vi "Inst_K2002.vi"(8 "error in":errorcluster, 10 "All Message Queues in":T1, 11 "Prueba31 in":refnum<class "Prueba05.lvclass">) -> (0 "error out":errorcluster)   [LabVIEW 2019, in "Prueba05.lvclass"]
uses:
  Prueba05.lvclass
  QMH/Message Queue/All Message Queues.ctl
  QMH/Message Queue/Message Cluster.ctl
  Prueba05.lvclass/Prueba05.ctl
  <vilib>/Utility/error.llb/Error Cluster From Error Code.vi
  QMH/Message Queue/Enqueue Message (Single).vi
  <vilib>/ErrorRing/Error Ring.xnode
  QMH/Message Queue/Message Queue.lvlib
  Instrumento/Keithley2002/Keithley2002.lvclass
panel:
  out "All States":string[](array[string])
  out "Actual State":string
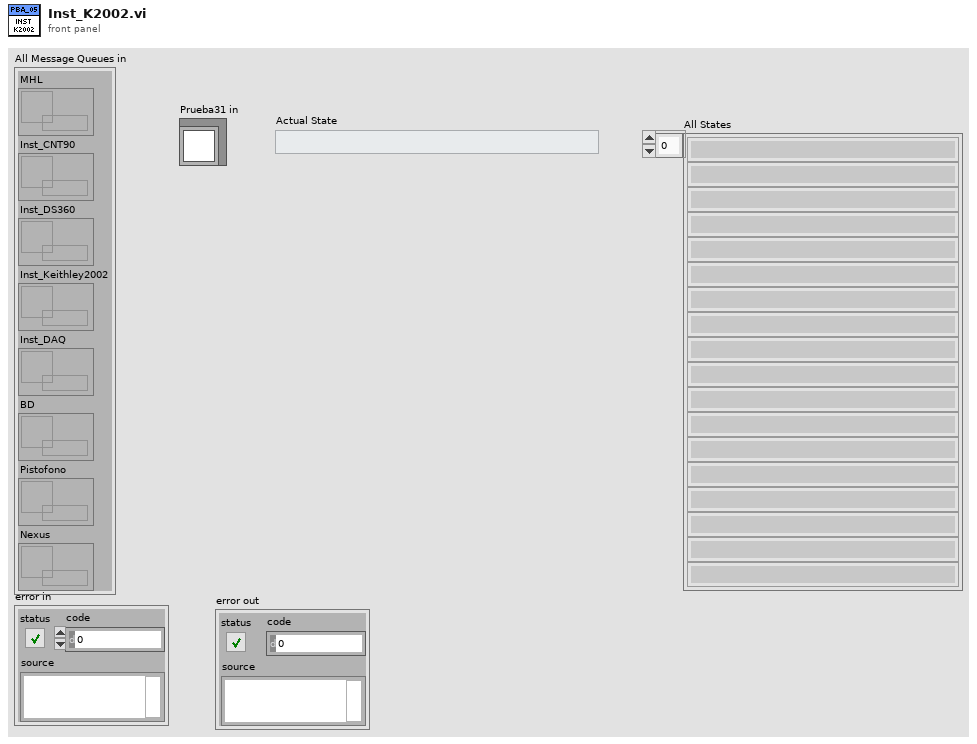
[diagram p1: front panel]
types:
  T1 = typedef "Message Queue.lvlib/All Message Queues.ctl" = cluster{"MHL":refnum<queue>, "Inst_CNT90":refnum<queue>, "Inst_DS360":refnum<queue>, "Inst_Keithley2002":refnum<queue>, "Inst_DAQ":refnum<queue>, "BD":refnum<queue>, "Pistofono":refnum<queue>, "Nexus":refnum<queue>}
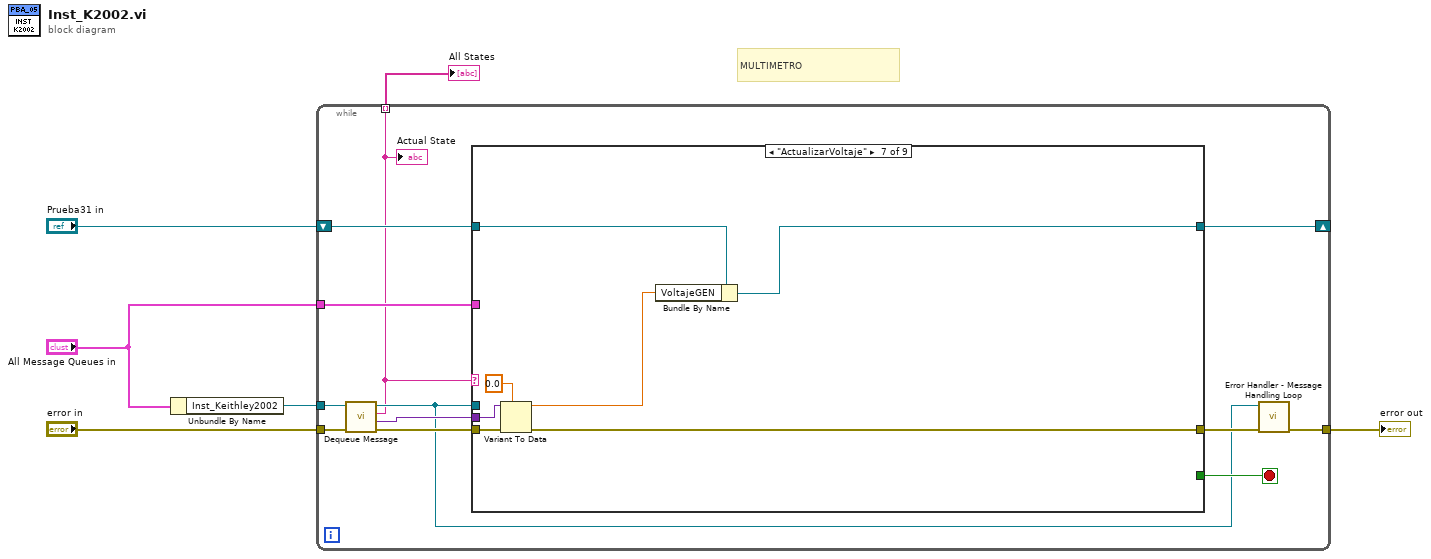
[diagram p0: block diagram]
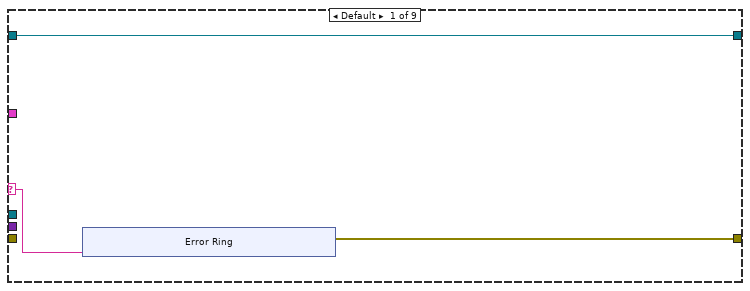
[diagram p2: hidden frame]
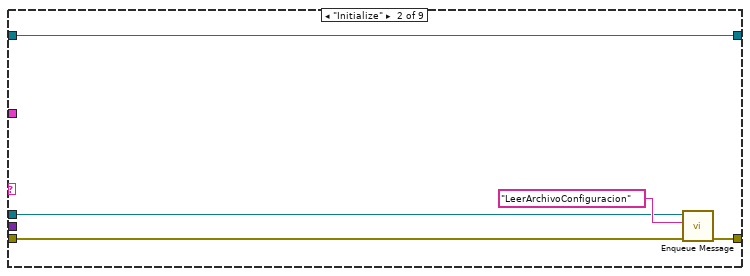
[diagram p3: hidden frame]
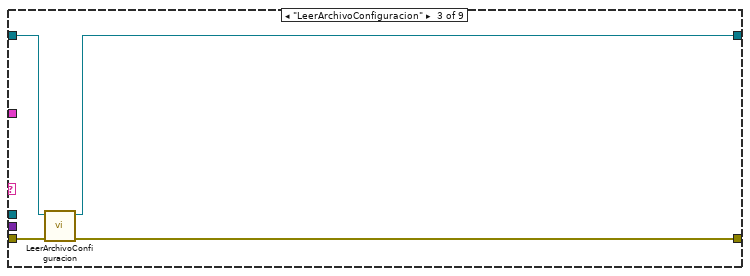
[diagram p4: hidden frame]
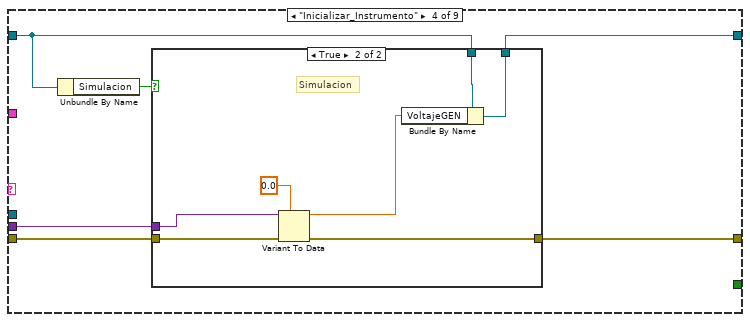
[diagram p5: hidden frame]
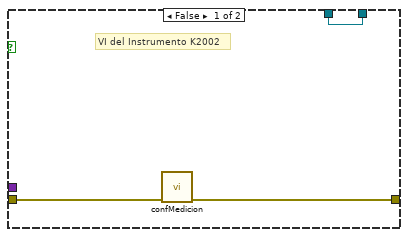
[diagram p6: hidden frame]
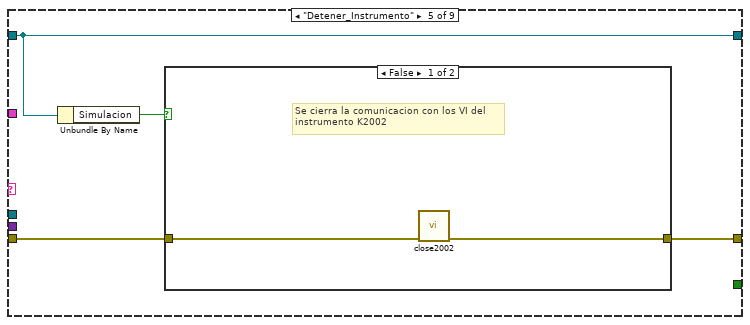
[diagram p7: hidden frame]
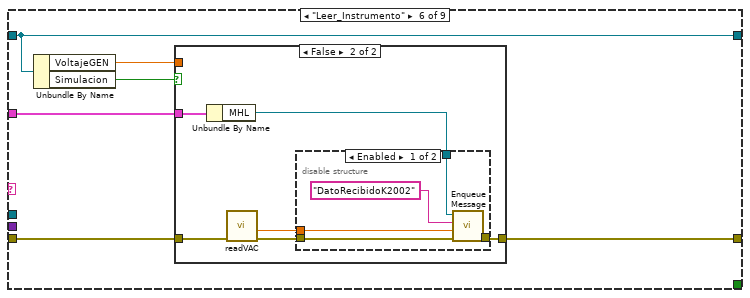
[diagram p9: hidden frame]
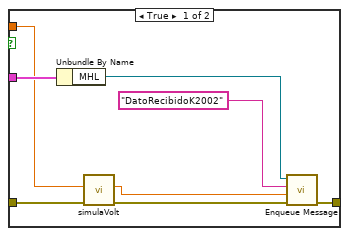
[diagram p10: hidden frame]
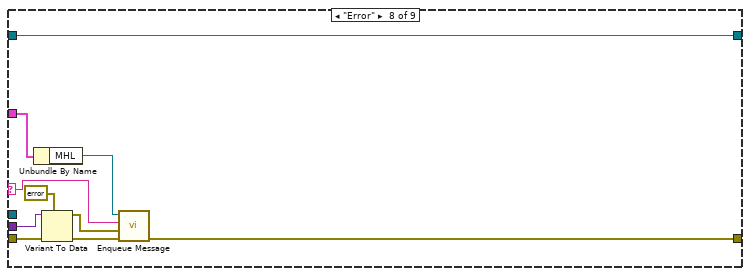
[diagram p12: hidden frame]
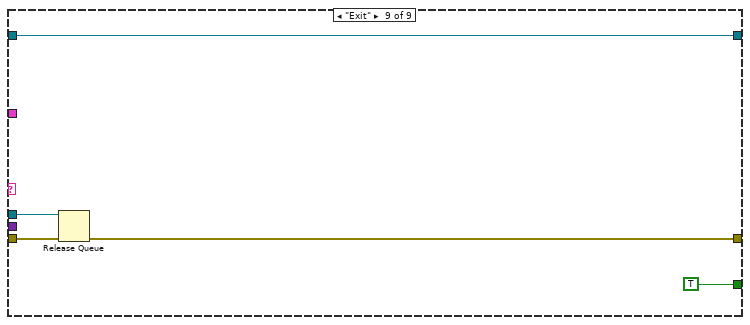
[diagram p13: hidden frame]
diagram:
  # "MULTIMETRO"
  n1 = Unbundle By Name("All Message Queues in") -> ("Inst_Keithley2002"=w4:refnum<queue>)
  n2 = while {
    tunnel: "error in" -> [w18]
    tunnel: w4 -> [w17]
    tunnel: "All Message Queues in" -> [w16]
    tunnel: [w9] -> w2
    shift-right: [w12] -> _
    shift-left: "Prueba31 in" -> [w15]
    tunnel: [w7] -> w1 mode=indexing
    stop <- w11 stop-if-true
    n3 = call "Dequeue Message.vi"("error in (no error)"=w18, "Message Queue"=w17) -> ("error out"=w13:errorcluster, "Message Data"=w14:variant, "Message"=w7:string, "dup Message Queue"=w8:refnum<queue>)  [unwired: 6 in]
    "Actual State" <- w7
    n4 = case shown="\"ActualizarVoltaje\"" w7 {
      selector: w7 -> [w21 _ _ _ _ _ _ w96 _]
      tunnel: w16 -> [_ _ _ _ _ w64 _ w95 _]
      tunnel: w15 -> [w19 w33 w34 w40 w56 w66 w88 w103 w105]
      tunnel: w8 -> [_ w29 _ _ _ _ _ _ w107]
      tunnel: w14 -> [_ _ _ w38 _ _ w90 w100 _]
      tunnel: w13 -> [_ w31 w36 w41 w54 w63 w92 w101 w108]
      tunnel: [w20 w30 w37 w43 w57 w62 w93 w98 w104] -> w10
      tunnel: [w19 w33 w35 w39 w56 w66 w89 w103 w105] -> w12
      tunnel: [_ _ _ _ _ _ _ _ TRUE] -> w11
      frame Default {
        n5 = xnode "Error Ring"("parameter 0"=w21) -> ("error out"=w20:errorcluster)
      }
      frame "Initialize" {
        n6 = call-poly "Enqueue Message.vi"("error in (no error)"=w31, "Message"="LeerArchivoConfiguracion", "Message Queue"=w29) -> ("error out"=w30:errorcluster)  [unwired: 7 in, 1 out]
      }
      frame "LeerArchivoConfiguracion" {
        n7 = call "LeerArchivoConfiguracion.vi"("error in"=w36, "Prueba05 in"=w34) -> ("error out"=w37:errorcluster, "Prueba05 out"=w35:refnum<class "Prueba05.lvclass">)  [unwired: 8 in]
      }
      frame "Inicializar_Instrumento" {
        n8 = Unbundle By Name(w40) -> ("Simulacion"=w42:bool)
        n9 = case shown="True" w42 {
          tunnel: [w46 w50] -> w43
          tunnel: w41 -> [w45 w53]
          tunnel: w40 -> [w44 w52]
          tunnel: [w44 w51] -> w39
          tunnel: w38 -> [_ w49]
          frame False {
            # "VI del Instrumento K2002"
            n10 = call "confMedicion.vi"("error in (no error)"=w45) -> ("error out"=w46:errorcluster)  [unwired: 9 in, 1 out]
          }
          frame True {
            # "Simulacion"
            n11 = Variant To Data(error in=w53, type=0.0, Variant=w49) -> (data=w47:dbl, error out=w50:errorcluster)
            n12 = Bundle By Name(cluster=w52, "VoltajeGEN"=w47) -> (w51:refnum<class "Prueba05.lvclass">)
          }
        }
      }
      frame "Detener_Instrumento" {
        n13 = Unbundle By Name(w56) -> ("Simulacion"=w55:bool)
        n14 = case shown="False" w55 {
          tunnel: [w59 w60] -> w57
          tunnel: w54 -> [w58 w60]
          frame False {
            # "Se cierra la comunicacion con los VI del\ninstrumento K2002"
            n15 = call "close2002.vi"("error in (no error)"=w58) -> ("error out"=w59:errorcluster)  [unwired: 9 in, 1 out]
          }
          frame True {
            # "Simulacion"
          }
        }
      }
      frame "Leer_Instrumento" {
        n16 = Unbundle By Name(w66) -> ("VoltajeGEN"=w61:dbl, "Simulacion"=w65:bool)
        n17 = case shown="False" w65 {
          tunnel: w64 -> [w74 w80]
          tunnel: [w71 w79] -> w62
          tunnel: w63 -> [w73 w77]
          tunnel: w61 -> [w68 _]
          frame True {
            n18 = Unbundle By Name(w74) -> ("MHL"=w70:refnum<queue>)
            n19 = call "simulaVolt.vi"("error in (no error)"=w73, "volt in"=w68) -> ("error out"=w72:errorcluster, "volt out"=w67:dbl)  [unwired: 7 in, 1 out]
            n20 = call-poly "Enqueue Message.vi"("error in (no error)"=w72, "Message Data"=w67, "Message"="DatoRecibidoK2002", "Message Queue"=w70) -> ("error out"=w71:errorcluster)  [unwired: 6 in, 1 out]
          }
          frame False {
            n21 = Unbundle By Name(w80) -> ("MHL"=w78:refnum<queue>)
            n22 = call "readVAC.vi"("error in (no error)"=w77) -> ("error out"=w76:errorcluster, "medicion"=w75:dbl)  [unwired: 7 in, 2 out]
            n23 = disable-structure shown="Enabled" {
              disable-tunnel: [w85 w86] -> w79
              disable-tunnel: w78 -> [w84 _]
              disable-tunnel: w76 -> [w82 w86]
              disable-tunnel: w75 -> [w81 _]
              frame Enabled {
                n24 = call-poly "Enqueue Message.vi"("error in (no error)"=w82, "Message Data"=w81, "Message"="DatoRecibidoK2002", "Message Queue"=w84) -> ("error out"=w85:errorcluster)  [unwired: 6 in, 1 out]
              }
              frame Disabled {
              }
            }
          }
        }
      }
      frame "ActualizarVoltaje" {
        n25 = Variant To Data(error in=w92, type=0.0, Variant=w90) -> (data=w87:dbl, error out=w93:errorcluster)
        n26 = Bundle By Name(cluster=w88, "VoltajeGEN"=w87) -> (w89:refnum<class "Prueba05.lvclass">)
      }
      frame "Error" {
        n27 = Unbundle By Name(w95) -> ("MHL"=w94:refnum<queue>)
        n28 = Variant To Data(error in=w101, type=errorcluster {"status"=FALSE, "code"=0, "source"=""} ("error constant"), Variant=w100) -> (data=w97:errorcluster, error out=w99:errorcluster)
        n29 = call-poly "Enqueue Message.vi"("error in (no error)"=w99, "Message Data"=w97, "Message"=w96, "Message Queue"=w94) -> ("error out"=w98:errorcluster)  [unwired: 6 in, 1 out]
      }
      frame "Exit" {
        n30 = Release Queue(queue=w107, error in (no error)=w108) -> (error out=w104:errorcluster)  [unwired: 1 in, 2 out]
      }
    }
    n31 = call "Error Handler - Message Handling Loop.vi"("error in (no error)"=w10, "Message Queue"=w8) -> ("dup error in"=w9:errorcluster)  [unwired: 8 in, 1 out]
  }
  "error out" <- w2
  "All States" <- w1
